vi "FPGA Main Image Processing - 7-7.vi"(9 "?":T1) -> ()   [LabVIEW 2017]
doc: "The myRIO v1.1 FPGA Shipping Personality. This personality contains support for:\n- 2 Analog Input Interrupt channel\n- 4 Digital Input Interrupt channel\n- 1 Timer\n- 1 Accelerometer\n- 1 Button\n- 4 LED\n- 10 Analog Input channels with 1 Sample\n- 6 Analog Output channels with 1 Sample\n- 40 Digital I/O channels with 1 Sample\n- 2 I2C channels\n- 4 Encoder channels\n- 6 PWM channels\n- 2 SPI channels"
uses:
  <vilib>/rvi/DataTransferAndStorage/Container/XNode/niFpgaContainer.xnode
  <vilib>/rvi/LocalResourceManager/LocalResourceManager.xnode
  SoC IP Library/SoC IP Library.lvlib
  <vilib>/rvi/Memory/Memory_Emulation/nirvimemoryFastEmulation.vi
  <vilib>/rvi/Memory/Memory_Emulation/nirvimemoryEmulation.vi
  <vilib>/rvi/interface/RandomDataEmulation/nirviRandomDataFpgaReadWriteTemplate.vi
  <vilib>/rvi/DataTransferAndStorage/Container/Common/niFpgaContainerGetUniqueNameForEmu.vi
  <vilib>/rvi/DataTransferAndStorage/Container/Common/niFpgaContainerSetEmuInfo.vi
  <vilib>/rvi/eio/common/nirviEmuReportErrorAndStop.vi
  SoC IP Library/Controls/Ocurrences.ctl
panel:
  out "SYS.RDY":bool
  # "Image Processing"
  # "System"
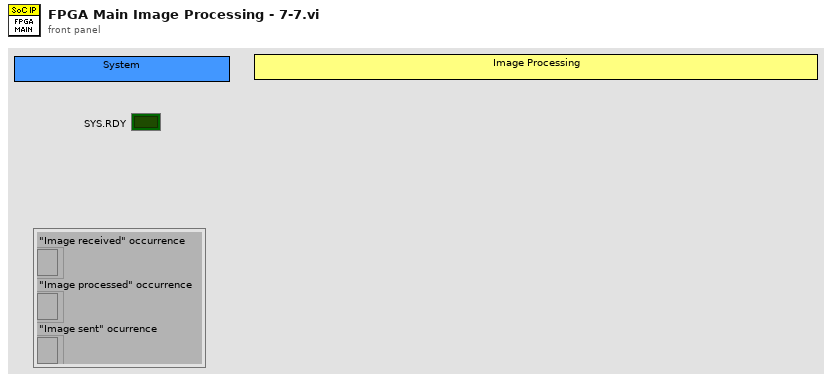
[diagram p1: front panel]
types:
  T1 = typedef "SoC IP Library.lvlib/Ocurrences.ctl" = cluster{"\"Image received\" occurrence":refnum<k4>, "\"Image processed\" occurrence":refnum<k4>, "\"Image sent\" ocurrence":refnum<k4>}
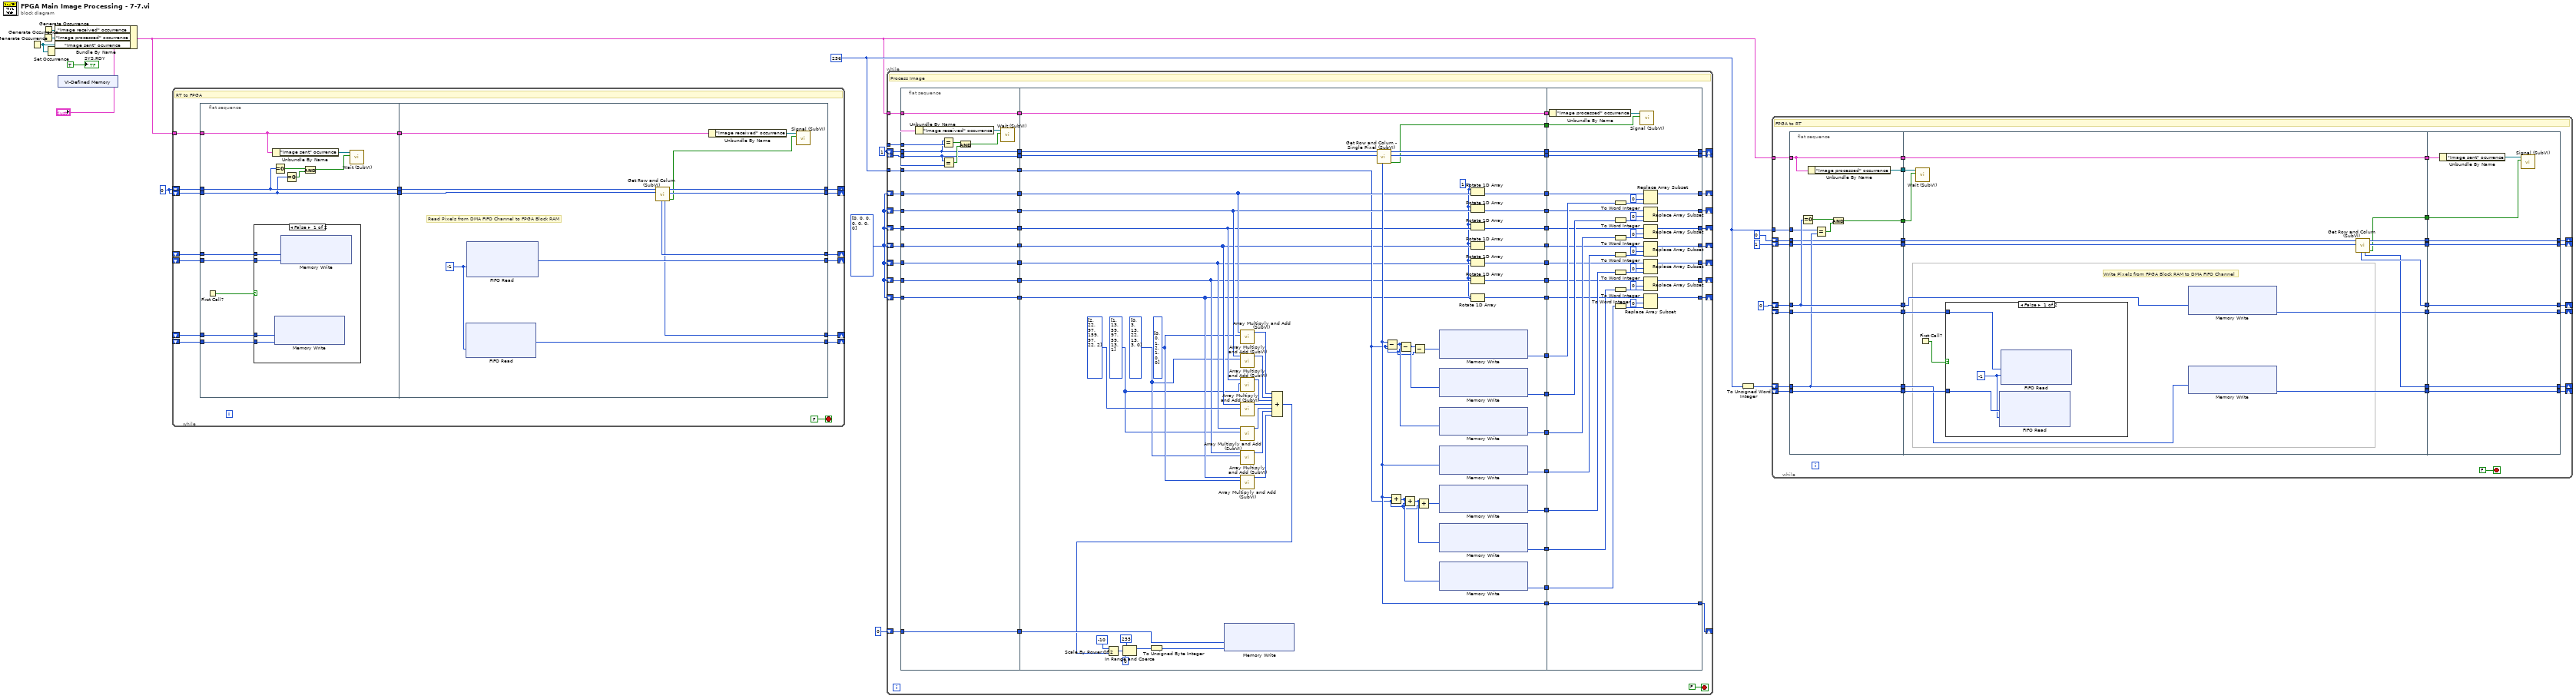
[diagram p0: block diagram]
diagram:
  w7 = u32 256 ("Dimension")
  w8 = i16[] [0, 0, 0, 0, 0, 0, 0]
  w10 = u8 1 ("Row Out")
  w13 = u8 0
  n1 = Generate Occurrence() -> (w6:refnum<k4>)
  n2 = Generate Occurrence() -> (w5:refnum<k4>)
  n3 = Generate Occurrence() -> (w4:refnum<k4>)
  n4 = Set Occurrence(w6) -> ()
  n5 = Bundle By Name(cluster="?", "\"Image received\" occurrence"=w4, "\"Image processed\" occurrence"=w5, "\"Image sent\" ocurrence"=w6) -> (w2:T1)
  n6 = xnode "VI-Defined Memory"() -> ()  [unwired: 1 out]
  n7 = while {
    shift-right: [w25] -> _
    shift-left: _ -> [w32]
    shift-right: [w19] -> _
    shift-left: _ -> [w31]
    shift-right: [w24] -> _
    shift-left: _ -> [w30]
    shift-right: [w28] -> _
    shift-left: _ -> [w29]
    shift-right: [w27] -> _
    shift-left: w13 -> [w23]
    shift-right: [w26] -> _
    shift-left: w13 -> [w22]
    tunnel: w2 -> [w18]
    stop <- FALSE stop-if-true
    # "RT to FPGA"
    n8 = flat-sequence {
      tunnel: w22 -> [w42]
      tunnel: w23 -> [w43]
      tunnel: w29 -> [w35]
      tunnel: w30 -> [w33]
      tunnel: w31 -> [w36]
      tunnel: w32 -> [w34]
      tunnel: [w43] -> w21
      tunnel: [w42] -> w20
      tunnel: w18 -> [w44]
      tunnel: [w44] -> w17
      tunnel: w21 -> [w56]
      tunnel: w20 -> [w55]
      tunnel: w17 -> [w52]
      tunnel: [w60] -> w19
      tunnel: [w59] -> w28
      tunnel: [w58] -> w27
      tunnel: [w57] -> w26
      tunnel: [w51] -> w25
      tunnel: [w50] -> w24
      frame #0 {
        n9 = First Call?() -> (First Call?: T/F=w37:bool)
        n10 = case shown="False" w37 {
          tunnel: w34 -> [w48 _]
          tunnel: w36 -> [w47 _]
          tunnel: w35 -> [w46 _]
          tunnel: w33 -> [w45 _]
          frame False {
            n11 = xnode ("Memory Write")("Address"=w45, "Data"=w46) -> ()  [unwired: 1 in, 1 out]
            n12 = xnode ("Memory Write")("Address"=w48, "Data"=w47) -> ()  [unwired: 1 in, 1 out]
          }
          frame True {
          }
        }
        n13 = Unbundle By Name(w44) -> ("\"Image sent\" ocurrence"=w39:refnum<k4>)
        n14 = Equal To 0?(x=w43) -> (x = 0?=w40:bool)
        n15 = Equal To 0?(x=w42) -> (x = 0?=w38:bool)
        n16 = And(x=w40, y=w38) -> (x .and. y?=w41:bool)
        n17 = call "Wait (SubVI).vi"("Wait? (T)"=w41, "Occurrence in"=w39) -> ()  [unwired: 10 in]
      }
      frame #1 {
        w53 = -1 ("Timeout")
        # "Read Pixels from DMA FIFO Channel to FPGA Block RAM"
        n18 = xnode ("FIFO Read")("Timeout"=w53) -> ("Element"=w59:u8)  [unwired: 1 in, 2 out]
        n19 = xnode ("FIFO Read")("Timeout"=w53) -> ("Element"=w60:u8)  [unwired: 1 in, 2 out]
        n20 = call "Get Row and Colum (SubVI).vi"("Colum In"=w55, "Row In"=w56) -> ("Last Pixel?"=w54:bool, "Colum Out"=w57:u8, "Row Out"=w58:u8, "Pixel B"=w50:u16, "Pixel A"=w51:u16)  [unwired: 5 in]
        n21 = Unbundle By Name(w52) -> ("\"Image received\" occurrence"=w49:refnum<k4>)
        n22 = call "Signal (SubVI).vi"("Set? (T)"=w54, "Occurrence in"=w49) -> ()  [unwired: 10 in]
      }
    }
  }
  n23 = while {
    tunnel: w2 -> [w114]
    shift-right: [w109] -> _
    shift-left: w10 -> [w104]
    shift-right: [w107] -> _
    shift-left: w10 -> [w105]
    tunnel: w7 -> [w102]
    shift-right: [w98] -> _
    shift-left: u32 0 ("Pixel") -> [w100]
    tunnel: w10 -> [w96]
    shift-right: [w91] -> _
    shift-left: w8 -> [w93]
    shift-right: [w90] -> _
    shift-left: w8 -> [w83]
    shift-right: [w89] -> _
    shift-left: w8 -> [w81]
    shift-right: [w88] -> _
    shift-left: w8 -> [w79]
    shift-right: [w87] -> _
    shift-left: w8 -> [w77]
    shift-right: [w86] -> _
    shift-left: w8 -> [w75]
    shift-right: [w85] -> _
    shift-left: w8 -> [w73]
    stop <- FALSE stop-if-true
    # "Process Image"
    n24 = flat-sequence {
      tunnel: w114 -> [w131]
      tunnel: [w131] -> w112
      tunnel: [w116] -> w106
      tunnel: w105 -> [w116]
      tunnel: w104 -> [w117]
      tunnel: [w117] -> w103
      tunnel: w102 -> [w130]
      tunnel: [w130] -> w101
      tunnel: w100 -> [w129]
      tunnel: [w129] -> w99
      tunnel: w96 -> [w128]
      tunnel: [w124] -> w94
      tunnel: w93 -> [w124]
      tunnel: [w123] -> w84
      tunnel: w83 -> [w123]
      tunnel: [w122] -> w82
      tunnel: w81 -> [w122]
      tunnel: [w121] -> w80
      tunnel: w79 -> [w121]
      tunnel: [w120] -> w78
      tunnel: w77 -> [w120]
      tunnel: [w119] -> w76
      tunnel: w75 -> [w119]
      tunnel: [w118] -> w74
      tunnel: w73 -> [w118]
      tunnel: [w187] -> w113
      tunnel: w112 -> [w187]
      tunnel: [w186] -> w111
      tunnel: [w185] -> w110
      tunnel: [w184] -> w108
      tunnel: w106 -> [w181]
      tunnel: w103 -> [w182]
      tunnel: w101 -> [w154]
      tunnel: w99 -> [w175]
      tunnel: [w162] -> w97
      tunnel: [w180] -> w95
      tunnel: w94 -> [w161]
      tunnel: [w153] -> w92
      tunnel: w84 -> [w160]
      tunnel: w82 -> [w159]
      tunnel: w80 -> [w146]
      tunnel: w78 -> [w145]
      tunnel: w76 -> [w144]
      tunnel: w74 -> [w143]
      tunnel: [w172] -> w72
      tunnel: [w171] -> w71
      tunnel: [w170] -> w70
      tunnel: [w169] -> w69
      tunnel: [w168] -> w68
      tunnel: [w167] -> w67
      tunnel: [w152] -> w66
      tunnel: [w151] -> w65
      tunnel: [w148] -> w64
      tunnel: [w147] -> w63
      tunnel: [w150] -> w62
      tunnel: [w149] -> w61
      tunnel: w113 -> [w228]
      tunnel: w111 -> [w226]
      tunnel: [w225] -> w109
      tunnel: w110 -> [w225]
      tunnel: w108 -> [w224]
      tunnel: [w224] -> w107
      tunnel: [w189] -> w98
      tunnel: w97 -> [w189]
      tunnel: w95 -> [w188]
      tunnel: w92 -> [w223]
      tunnel: [w220] -> w91
      tunnel: [w217] -> w90
      tunnel: [w207] -> w89
      tunnel: [w206] -> w88
      tunnel: [w205] -> w87
      tunnel: [w204] -> w86
      tunnel: [w203] -> w85
      tunnel: w72 -> [w202]
      tunnel: w71 -> [w201]
      tunnel: w70 -> [w197]
      tunnel: w69 -> [w198]
      tunnel: w68 -> [w199]
      tunnel: w67 -> [w200]
      tunnel: w66 -> [w196]
      tunnel: w65 -> [w191]
      tunnel: w64 -> [w194]
      tunnel: w63 -> [w195]
      tunnel: w62 -> [w192]
      tunnel: w61 -> [w193]
      frame #0 {
        n25 = Unbundle By Name(w131) -> ("\"Image received\" occurrence"=w132:refnum<k4>)
        n26 = Equal?(x=w116, y=w128) -> (x = y?=w127:bool)
        n27 = Equal?(x=w117, y=w128) -> (x = y?=w126:bool)
        n28 = And(x=w127, y=w126) -> (x .and. y?=w125:bool)
        n29 = call "Wait (SubVI).vi"("Wait? (T)"=w125, "Occurrence in"=w132) -> ()  [unwired: 10 in]
      }
      frame #1 {
        w142 = 1 ("n")
        w140 = i16[] [0, 3, 13, 22, 13, 3, 0]
        w139 = i16[] [1, 13, 59, 97, 59, 13, 1]
        w141 = i16[] [0, 0, 1, 2, 1, 0, 0]
        n30 = call "Array Multipyly and Add (SubVI).vi"("Array 2"=w141, "Array"=w161) -> ("Numeric"=w157:i32)  [unwired: 9 in]
        n31 = call "Array Multipyly and Add (SubVI).vi"("Array 2"=w140, "Array"=w160) -> ("Numeric"=w156:i32)  [unwired: 9 in]
        n32 = call "Array Multipyly and Add (SubVI).vi"("Array 2"=w139, "Array"=w159) -> ("Numeric"=w138:i32)  [unwired: 9 in]
        n33 = call "Array Multipyly and Add (SubVI).vi"("Array 2"=i16[] [2, 22, 97, 159, 97, 22, 2], "Array"=w146) -> ("Numeric"=w134:i32)  [unwired: 9 in]
        n34 = call "Array Multipyly and Add (SubVI).vi"("Array 2"=w139, "Array"=w145) -> ("Numeric"=w135:i32)  [unwired: 9 in]
        n35 = call "Array Multipyly and Add (SubVI).vi"("Array 2"=w140, "Array"=w144) -> ("Numeric"=w136:i32)  [unwired: 9 in]
        n36 = call "Array Multipyly and Add (SubVI).vi"("Array 2"=w141, "Array"=w143) -> ("Numeric"=w137:i32)  [unwired: 9 in]
        n37 = Compound Arithmetic op=ADD(w157, w156, w138, w134, w135, w136, w137) -> (w133:i32)
        n38 = Scale By Power Of 2(n=i16 -10, x=w133) -> (x*2^n=w177:i32)
        n39 = In Range and Coerce(upper limit=i16 255, x=w177, lower limit=i16 0) -> (coerced(x)=w178:i32)  [unwired: 1 out]
        n40 = To Unsigned Byte Integer(number=w178) -> (unsigned 8bit integer=w176:u8)
        n41 = xnode ("Memory Write")("Address"=w175, "Data"=w176) -> ()  [unwired: 1 in, 1 out]
        n42 = call "Get Row and Colum - Single Pixel (SubVI).vi"("Colum In"=w182, "Row In"=w181) -> ("Last Pixel?"=w180:bool, "Colum Out"=w185:u8, "Row Out"=w184:u8, "Pixel"=w162:u16)  [unwired: 6 in]
        n43 = Subtract(x=w162, y=w154) -> (x-y=w173:u32)
        n44 = Add(x=w162, y=w154) -> (x+y=w163:u32)
        n45 = Subtract(x=w173, y=w154) -> (x-y=w174:u32)
        n46 = Add(x=w163, y=w154) -> (x+y=w164:u32)
        n47 = Subtract(x=w174, y=w154) -> (x-y=w166:u32)
        n48 = Add(x=w164, y=w154) -> (x+y=w165:u32)
        n49 = xnode ("Memory Write")("Address"=w166) -> ("Data"=w186:u8)  [unwired: 1 in, 1 out]
        n50 = xnode ("Memory Write")("Address"=w174) -> ("Data"=w172:u8)  [unwired: 1 in, 1 out]
        n51 = xnode ("Memory Write")("Address"=w173) -> ("Data"=w171:u8)  [unwired: 1 in, 1 out]
        n52 = xnode ("Memory Write")("Address"=w162) -> ("Data"=w167:u8)  [unwired: 1 in, 1 out]
        n53 = xnode ("Memory Write")("Address"=w165) -> ("Data"=w168:u8)  [unwired: 1 in, 1 out]
        n54 = xnode ("Memory Write")("Address"=w164) -> ("Data"=w169:u8)  [unwired: 1 in, 1 out]
        n55 = xnode ("Memory Write")("Address"=w163) -> ("Data"=w170:u8)  [unwired: 1 in, 1 out]
        n56 = Rotate 1D Array(1:w161, 2:w142) -> (0:w153:i16[])
        n57 = Rotate 1D Array(1:w160, 2:w142) -> (0:w152:i16[])
        n58 = Rotate 1D Array(1:w159, 2:w142) -> (0:w151:i16[])
        n59 = Rotate 1D Array(1:w146, 2:w142) -> (0:w150:i16[])
        n60 = Rotate 1D Array(1:w145, 2:w142) -> (0:w149:i16[])
        n61 = Rotate 1D Array(1:w144, 2:w142) -> (0:w148:i16[])
        n62 = Rotate 1D Array(1:w143, 2:w142) -> (0:w147:i16[])
      }
      frame #2 {
        n63 = Unbundle By Name(w228) -> ("\"Image processed\" occurrence"=w227:refnum<k4>)
        n64 = To Word Integer(number=w226) -> (16bit integer=w222:i16)
        n65 = To Word Integer(number=w202) -> (16bit integer=w219:i16)
        n66 = To Word Integer(number=w201) -> (16bit integer=w216:i16)
        n67 = To Word Integer(number=w200) -> (16bit integer=w214:i16)
        n68 = To Word Integer(number=w199) -> (16bit integer=w212:i16)
        n69 = To Word Integer(number=w198) -> (16bit integer=w210:i16)
        n70 = To Word Integer(number=w197) -> (16bit integer=w190:i16)
        n71 = call "Signal (SubVI).vi"("Set? (T)"=w188, "Occurrence in"=w227) -> ()  [unwired: 10 in]
        n72 = Replace Array Subset(array=w223, new element=w222, index=0) -> (w220:i16[])
        n73 = Replace Array Subset(array=w196, new element=w219, index=0) -> (w217:i16[])
        n74 = Replace Array Subset(array=w191, new element=w216, index=0) -> (w207:i16[])
        n75 = Replace Array Subset(array=w192, new element=w214, index=0) -> (w206:i16[])
        n76 = Replace Array Subset(array=w193, new element=w212, index=0) -> (w205:i16[])
        n77 = Replace Array Subset(array=w194, new element=w210, index=0) -> (w204:i16[])
        n78 = Replace Array Subset(array=w195, new element=w190, index=0) -> (w203:i16[])
      }
    }
  }
  n79 = To Unsigned Word Integer(number=w7) -> (unsigned 16bit integer=w9:u16)
  n80 = while {
    shift-right: [w256] -> _
    shift-left: u16 0 -> [w260]
    shift-right: [w255] -> _
    shift-left: w9 -> [w259]
    shift-right: [w258] -> _
    shift-left: u8 0 -> [w254]
    shift-right: [w257] -> _
    shift-left: u8 1 ("Colum Out") -> [w253]
    shift-right: [w244] -> _
    shift-left: _ -> [w240]
    shift-right: [w242] -> _
    shift-left: _ -> [w238]
    tunnel: w7 -> [w234]
    tunnel: w2 -> [w233]
    stop <- FALSE stop-if-true
    # "FPGA to RT"
    n81 = flat-sequence {
      tunnel: w253 -> [w264]
      tunnel: w254 -> [w265]
      tunnel: w259 -> [w267]
      tunnel: w260 -> [w268]
      tunnel: [w268] -> w252
      tunnel: [w267] -> w251
      tunnel: [w270] -> w241
      tunnel: w240 -> [w270]
      tunnel: [w269] -> w239
      tunnel: w238 -> [w269]
      tunnel: [w266] -> w237
      tunnel: [w265] -> w236
      tunnel: [w264] -> w235
      tunnel: w234 -> [w263]
      tunnel: w233 -> [w262]
      tunnel: [w262] -> w232
      tunnel: [w261] -> w230
      tunnel: w252 -> [w279]
      tunnel: w251 -> [w278]
      tunnel: [w289] -> w250
      tunnel: [w288] -> w249
      tunnel: [w287] -> w248
      tunnel: [w286] -> w247
      tunnel: [w285] -> w246
      tunnel: [w284] -> w245
      tunnel: [w283] -> w243
      tunnel: w241 -> [w282]
      tunnel: w239 -> [w281]
      tunnel: w237 -> [w275]
      tunnel: w236 -> [w277]
      tunnel: w235 -> [w276]
      tunnel: w232 -> [w274]
      tunnel: [w274] -> w231
      tunnel: w230 -> [w273]
      tunnel: [w298] -> w255
      tunnel: [w299] -> w256
      tunnel: [w300] -> w257
      tunnel: [w301] -> w258
      tunnel: w250 -> [w301]
      tunnel: w249 -> [w300]
      tunnel: w248 -> [w299]
      tunnel: w247 -> [w298]
      tunnel: w246 -> [w295]
      tunnel: [w297] -> w244
      tunnel: w245 -> [w297]
      tunnel: [w296] -> w242
      tunnel: w243 -> [w296]
      tunnel: w231 -> [w294]
      frame #0 {
        n82 = Equal To 0?(x=w268) -> (x = 0?=w271:bool)
        n83 = Unbundle By Name(w262) -> ("\"Image processed\" occurrence"=w261:refnum<k4>)
        n84 = Equal?(x=w263, y=w267) -> (x = y?=w272:bool)
        n85 = And(x=w271, y=w272) -> (x .and. y?=w266:bool)
      }
      frame #1 {
        # "Write Pixels from FPGA Block RAM to DMA FIFO Channel"
        n86 = call "Wait (SubVI).vi"("Wait? (T)"=w275, "Occurrence in"=w273) -> ()  [unwired: 10 in]
        n87 = First Call?() -> (First Call?: T/F=w280:bool)
        n88 = case shown="False" w280 {
          tunnel: w282 -> [w292 _]
          tunnel: w281 -> [w291 _]
          frame False {
            w290 = -1 ("Timeout")
            n89 = xnode ("FIFO Read")("Element"=w291, "Timeout"=w290) -> ()  [unwired: 1 in, 2 out]
            n90 = xnode ("FIFO Read")("Element"=w292, "Timeout"=w290) -> ()  [unwired: 1 in, 2 out]
          }
          frame True {
          }
        }
        n91 = xnode ("Memory Write")("Address"=w279) -> ("Data"=w284:u8)  [unwired: 1 in, 1 out]
        n92 = xnode ("Memory Write")("Address"=w278) -> ("Data"=w283:u8)  [unwired: 1 in, 1 out]
        n93 = call "Get Row and Colum (SubVI).vi"("Colum In"=w276, "Row In"=w277) -> ("Last Pixel?"=w285:bool, "Colum Out"=w288:u8, "Row Out"=w289:u8, "Pixel B"=w286:u16, "Pixel A"=w287:u16)  [unwired: 5 in]
      }
      frame #2 {
        n94 = Unbundle By Name(w294) -> ("\"Image sent\" ocurrence"=w293:refnum<k4>)
        n95 = call "Signal (SubVI).vi"("Set? (T)"=w295, "Occurrence in"=w293) -> ()  [unwired: 10 in]
      }
    }
  }
  "SYS.RDY" <- TRUE
